vi "Init Wrapper.vi"(6 "DLL Directory":path, 8 "error in":errorcluster, 10 "JPG (F)":bool, 11 "PNG (F)":bool) -> (0 "error out":errorcluster, 3 "Flags Successfully Initialised":i32 format="%.0x")   [LabVIEW 2015, in "LibSDL2_Image.lvlib"]
doc: "Note that in order for this call to work properly the the CurrentDirectory needs to be set so that the DLLs can be found in the correct place."
uses:
  LibSDL2_Image.lvlib
  Win32 Util/Win32 Util.lvlib
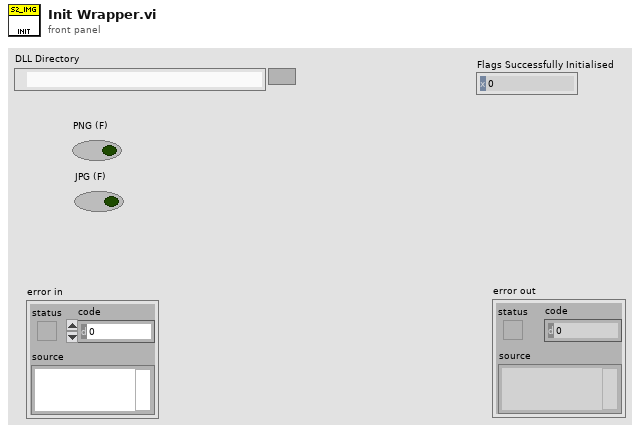
[diagram p1: front panel]
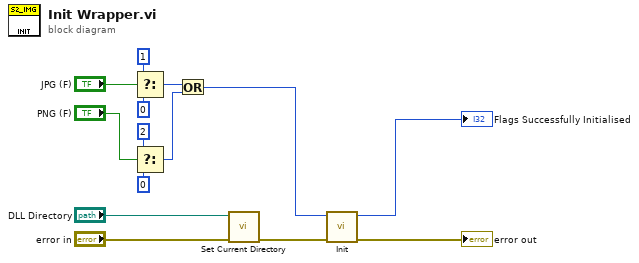
[diagram p0: block diagram]
diagram:
  n1 = Select(t=1, s="JPG (F)", f=0) -> (s? t:f=w11:i32)
  n2 = Select(t=2, s="PNG (F)", f=0) -> (s? t:f=w7:i32)
  n3 = Or(x=w11, y=w7) -> (x .or. y?=w6:i32)
  n4 = call "Set Current Directory.vi"("error in (no error)"="error in", "Path"="DLL Directory") -> ("error out"=w3:errorcluster)  [unwired: 9 in]
  n5 = call "Init.vi"("error in"=w3, "Flags"=w6) -> ("error out"=→"error out":errorcluster, "Flags Successfully Initialised"=→"Flags Successfully Initialised":i32)  [unwired: 8 in]
